vi "Compare DMA.vi"(1 "Target bitfile DMA in":T1[](array[typedef]) {"Data Type" format="%.0x"}, 2 "Reference bitfile DMA in":T1[](array[typedef]) {"Data Type" format="%.0x"}) -> (0 "Equal ?":bool)   [LabVIEW 2026, in "FPGA Addon Bitfile Reload Unit Tests.lvclass"]
uses:
  FPGA Addon Bitfile Reload Unit Tests.lvclass
  Addon/Addon Shared/Types/DMA Information.ctl
  Addon/Addon Shared/FPGA Addon Shared.lvlib
  Addon/Addon Shared/Types/FPGA Addon Data Type.ctl
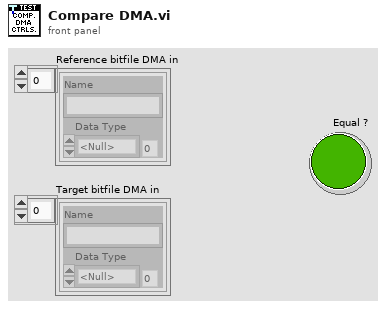
[diagram p1: front panel]
types:
  T1 = typedef "FPGA Addon Shared.lvlib/DMA Information.ctl" = cluster{"Name":string, "Data Type":T2}
  T2 = typedef "FPGA Addon Shared.lvlib/FPGA Addon Data Type.ctl" = enum8{"<Null>", "I8", "I16", "I32", "I64", "U8", "U16", "U32", "U64", "SGL", "Boolean", "Analog PWM In Settings", "Analog PWM In", "Digital PWM In Settings", "Digital PWM In", "Digital PWM Out", "Sine Out", "FXP", "FXP+/-24.5", "FXP+/-16.5", "FXP+/-32.8", "FXP+/-64.32", "FXP+/-16.7", "FXP+/-20.5", "FXP+/-27.5", "FXP+/-32.16", "FXP+16.3", "FXP+18.3", "Digital Static In", "Digital Static Out", "Digital Static In Settings", "Digital WSS Out", "Quad Encoder Settings", "Quad Encoder In", "Group"}
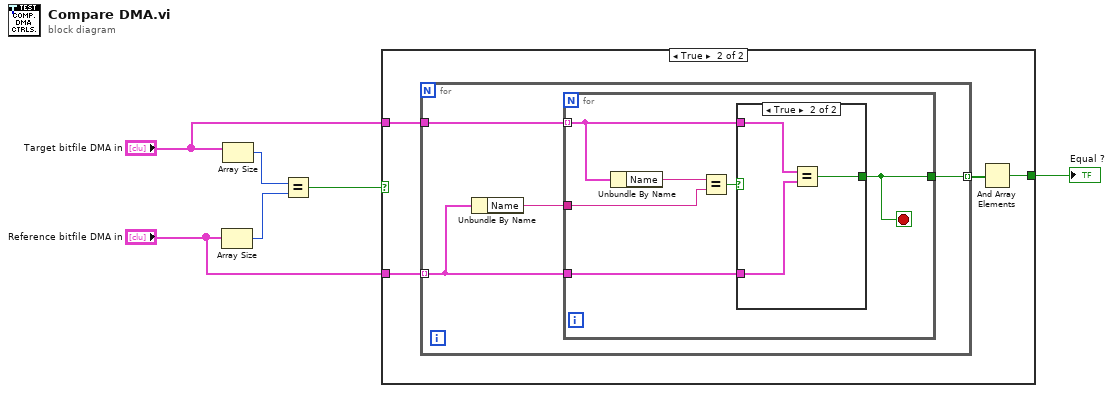
[diagram p0: block diagram]
diagram:
  n1 = Array Size(array="Reference bitfile DMA in") -> (size(s)=w6:i32)
  n2 = Array Size(array="Target bitfile DMA in") -> (size(s)=w5:i32)
  n3 = Equal?(x=w5, y=w6) -> (x = y?=w3:bool)
  n4 = case shown="True" w3 {
    tunnel: "Target bitfile DMA in" -> [_ w9]
    tunnel: "Reference bitfile DMA in" -> [_ w10]
    tunnel: [_ w7] -> w4
    frame False {
    }
    frame True {
      n5 = for {
        tunnel: w10 -> [w12] mode=indexing
        tunnel: w9 -> [w14]
        tunnel: [w11] -> w8 mode=indexing
        n6 = Unbundle By Name(w12) -> ("Name"=w13:string)
        n7 = for {
          tunnel: w14 -> [w17] mode=indexing
          tunnel: w13 -> [w19]
          tunnel: w12 -> [w16]
          tunnel: [w15] -> w11
          stop <- w15 stop-if-true
          n8 = Unbundle By Name(w17) -> ("Name"=w20:string)
          n9 = Equal?(x=w20, y=w19) -> (x = y?=w18:bool)
          n10 = case shown="True" w18 {
            tunnel: w17 -> [_ w23]
            tunnel: w16 -> [_ w22]
            tunnel: [_ w21] -> w15
            frame False {
            }
            frame True {
              n11 = Equal?(x=w23, y=w22) -> (x = y?=w21:bool)
            }
          }
        }
      }
      n12 = And Array Elements(Boolean array=w8) -> (logical AND=w7:bool)
    }
  }
  "Equal ?" <- w4
